vi "Select Cartridge.vi"(1 "Relative Address in":u32 format="%.0x", 2 "Cartridge band":u32) -> (0 "Relative Address out":u32 format="%.0x")   [LabVIEW 2017]
panel:
  # "ALMA Monitor and Control Bus\nSelect Cartridge"
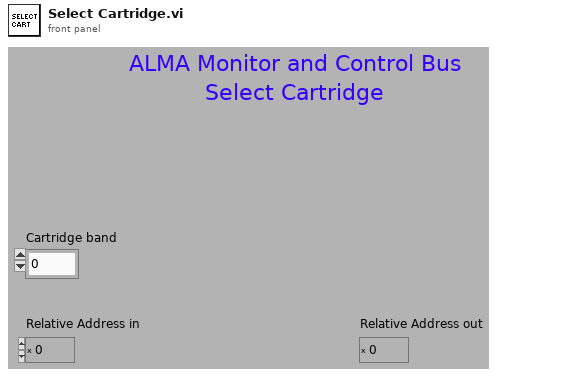
[diagram p1: front panel]
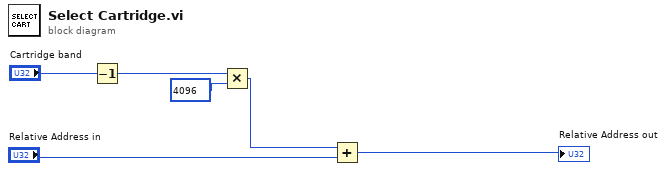
[diagram p0: block diagram]
diagram:
  n1 = Decrement(x="Cartridge band") -> (x-1=w1:u32)
  n2 = Multiply(x=w1, y=u32 4096) -> (x*y=w2:u32)
  n3 = Add(x=w2, y="Relative Address in") -> (x+y=→"Relative Address out":u32)
